vi "Fourier Synthesis.vi"() -> ()   [LabVIEW 2019]
uses:
  <vilib>/Analysis/2dsp.llb/Real FFT.vi
  <vilib>/measure/NI_MABase.lvlib
  <vilib>/Analysis/NI_AALPro.lvlib
panel:
  in  "Display Tab":enum32{"Re - Im", "Magnitude"}(tab)
  out "Real":cluster{"Integers Out":i32[], dbl[]}(graph)
  out "Imaginary":cluster{"Integers Out":i32[], dbl[]}(graph)
  out "Phase":cluster{i32[], dbl[]}(graph)
  out "Magnitudes":cluster{i32[], dbl[]}(graph)
  in  "Rectify":bool
  in  "Amplitude":dbl=1.0 min=-10.0 max=10.0 step=0.1
  in  "Offset":dbl min=-10.0 max=10.0 step=0.1
  out "Summed curves":waveform(dbl)[](graph)
  out "Individual curves":waveform(dbl)[](graph)=[{"t0"=timestamp(21.7 s since 1904-01-01), "dt"=0.0001, "Y"=array[3000 elements]}]
  out "Original":waveform(dbl)(graph)={"t0"=timestamp(0 s since 1904-01-01), "dt"=0.0001, "Y"=array[3000 elements]}
  in  "Stop Button":bool
  in  "Signal Type":u16(ring)=2 items=["Sine Wave", "Triangle Wave", "Square Wave", "Sawtooth Wave"]
  in  "No. of coefficients":i32(slide) min=0 max=100 step=1 scale=0.0..20.0
  in  "Phase [Deg]":dbl=180.0 min=-360.0 max=360.0 step=0.1
  in  "Duty Cycle [%]":dbl=50.0 min=0.0 max=100.0 step=1.0
  # "Fourier Synthesis Example"
  # "McClellan et al., DSP First, 2nd ed.\nCh 3-5: Fourier series"
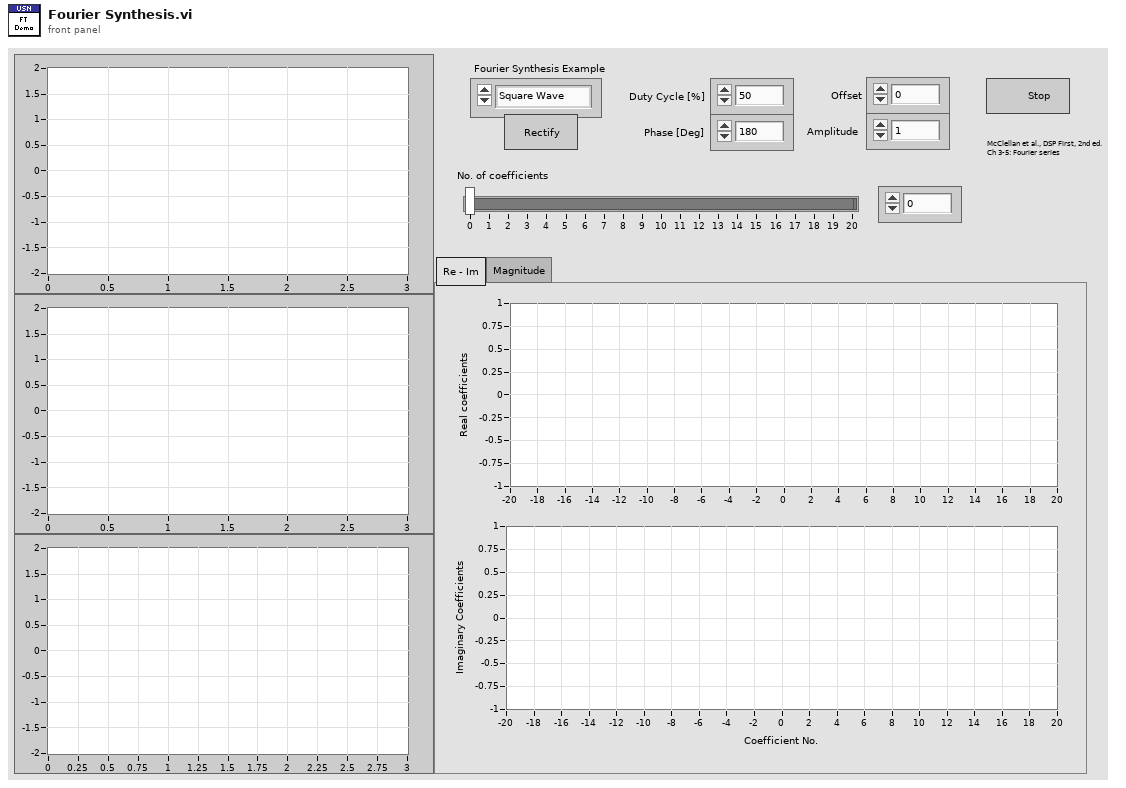
[diagram p1: front panel]
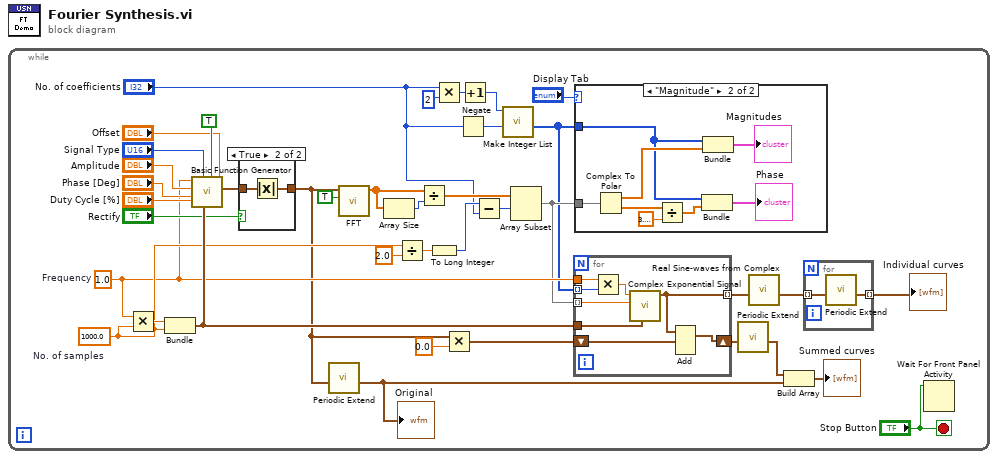
[diagram p0: block diagram]
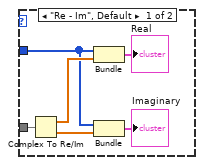
[diagram p2: hidden frame]
diagram:
  n1 = while {
    stop <- "Stop Button" stop-if-true
    w19 = 1.0  # Frequency
    w23 = 1000.0  # No. of samples
    n2 = Multiply(x=w19, y=w23) -> (x*y=w39:dbl)
    n3 = Bundle(w39, "No. of samples"=w23) -> (w38:cluster{dbl, "No. of samples":dbl})  [unwired: 1 out]
    n4 = call <vilib>:"Basic Function Generator.vi"("offset"="Offset", "square wave duty cycle (%)"="Duty Cycle [%]", "reset signal"=TRUE ("Reset signal"), "sampling info"=w38, "signal type"="Signal Type", "phase"="Phase [Deg]", "amplitude"="Amplitude", "frequency"=w19) -> ("signal out"=w28:waveform(dbl))  [unwired: 1 in, 2 out]
    n5 = case shown="True" "Rectify" {
      tunnel: w28 -> [w56 w58]
      tunnel: [w56 w57] -> w8
      frame False {
      }
      frame True {
        n6 = Absolute Value(x=w58) -> (abs(x)=w57:waveform(dbl))
      }
    }
    n7 = call "Periodic Extend.vi"("Waveform in"=w8) -> ("Waveform out"=w7:waveform(dbl))  [unwired: 8 in, 2 out]
    "Original" <- w7
    n8 = call-poly <vilib>:"FFT.vi"("shift?"=TRUE, "X"=w8) -> ("FFT {X}"=w37:cdb[])  [unwired: 1 in, 8 out]
    n9 = Array Size(array=w37) -> (size(s)=w25:i32)
    n10 = Divide(x=w23, y=2.0) -> (x/y=w24:dbl)
    n11 = Divide(x=w37, y=w25) -> (x/y=w18:cdb[])
    n12 = To Long Integer(number=w24) -> (32bit integer=w12:i32)
    n13 = Multiply(x="No. of coefficients", y=2) -> (x*y=w17:i32)
    n14 = Multiply(x=w8, y=0.0) -> (x*y=w14:waveform(dbl))
    n15 = Negate(x="No. of coefficients") -> (-x=w6:i32)
    n16 = Increment(x=w17) -> (x+1=w4:i32)
    n17 = Subtract(x=w12, y="No. of coefficients") -> (x-y=w13:i32)
    n18 = call "Make Integer List.vi"("Start"=w6, "No. of elements"=w4) -> ("Integers Out"=w5:i32[])  [unwired: 8 in, 1 out]
    n19 = Array Subset(array=w18, index=w13) -> (w10:cdb[])  [unwired: 1 in]
    n20 = for {
      tunnel: w38 -> [w65]
      shift-right: [w66] -> w21
      shift-left: w14 -> [w60]
      tunnel: w19 -> [w62]
      tunnel: w10 -> [w64] mode=indexing
      tunnel: w5 -> [w63] mode=indexing
      tunnel: [w59] -> w3 mode=indexing
      n21 = Multiply(x=w62, y=w63) -> (x*y=w61:dbl)
      n22 = call "Complex Exponential Signal.vi"("sampling info"=w65, "amplitude"=w64, "frequency"=w61) -> ("signal out"=w59:waveform(cdb))  [unwired: 7 in, 1 out]
      n23 = Add(1:w60, 2:w59) -> (0:w66:waveform(cdb))  [unwired: 1 in, 1 out]
    }
    n24 = case shown="\"Magnitude\"" "Display Tab" {
      tunnel: w5 -> [w42 w50]
      tunnel: w10 -> [w44 w52]
      frame "Re - Im", Default {
        n25 = Complex To Re/Im(x + iy=w44) -> (x=w43:dbl[], y=w45:dbl[])
        n26 = Bundle("Integers Out"=w42, w43) -> (→"Real":cluster{"Integers Out":i32[], dbl[]})  [unwired: 1 in]
        n27 = Bundle("Integers Out"=w42, w45) -> (→"Imaginary":cluster{"Integers Out":i32[], dbl[]})  [unwired: 1 in]
      }
      frame "Magnitude" {
        n28 = Complex To Polar(r * e^(i*theta)=w52) -> (r=w53:dbl[], theta=w48:dbl[])
        n29 = Divide(x=w48, y=3.141592653589793) -> (x/y=w46:dbl[])
        n30 = Bundle("Integers Out"=w50, w46) -> (→"Phase":cluster{"Integers Out":i32[], dbl[]})  [unwired: 1 in]
        n31 = Bundle("Integers Out"=w50, w53) -> (→"Magnitudes":cluster{"Integers Out":i32[], dbl[]})  [unwired: 1 in]
      }
    }
    n32 = call "Periodic Extend.vi"("Waveform in"=w21) -> ("Waveform out"=w20:waveform(dbl))  [unwired: 8 in, 2 out]
    n33 = call "Real Sine-waves from Complex.vi"("Complex Waveforms In"=w3) -> ("Real Waveforms Out"=w2:waveform(dbl)[])  [unwired: 9 in, 1 out]
    n34 = Build Array(w20, w7) -> (→"Summed curves":waveform(dbl)[])
    n35 = for {
      tunnel: w2 -> [w55] mode=indexing
      tunnel: [w54] -> w22 mode=indexing
      n36 = call "Periodic Extend.vi"("Waveform in"=w55) -> ("Waveform out"=w54:waveform(dbl))  [unwired: 8 in, 2 out]
    }
    "Individual curves" <- w22
    n37 = Wait For Front Panel Activity(3:"Stop Button") -> ()  [unwired: 3 out]
  }
